vi "Magazine control.vi"(0 "Intake power":dbl, 1 "Magazine power":dbl, 2 "Magazine Recovery Power":dbl, 3 "Magazine Intake power":dbl, 4 "Flywheel power":dbl, 5 "Idle flywheel power":dbl, 7 "Intake sensor":bool, 8 "Intake":bool, 10 "Shoot":bool, 11 "Outtake sensor":bool, 12 "Emergency force state":T1(ring)=enum."Nil", 13 "Initial state":T1(ring)=enum."Idle") -> (14 "Intake":dbl, 15 "Magazine":dbl, 18 "Flywheel":dbl)   [LabVIEW 2019]
panel:
  out "State":T1(ring)=enum."I-mode tweak from intake"
  # "If both (or neither) are false, the magazine goes into the idle state."
  # "These inputs can interrupt the current state."
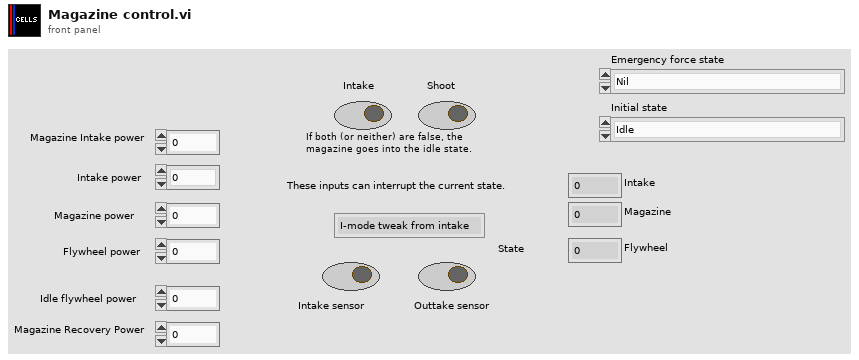
[diagram p1: front panel]
types:
  T1 = enum16{"I-mode wait for cell", "I-mode move to intake", "I-mode tweak from intake", "I-mode move cells in", "Idle", "O-mode move to outtake", "O-mode wait to shoot", "Recover from full magazine", "O-mode shoot", "Nil", "O-mode move to outtake w/o shoot"}
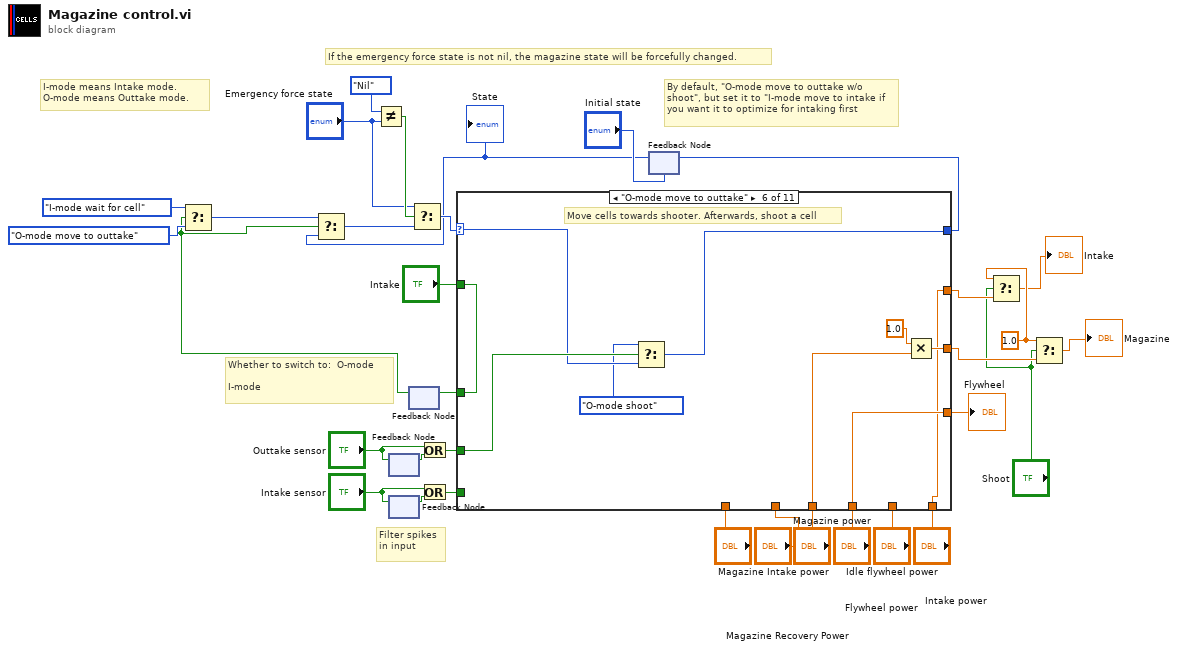
[diagram p0: block diagram]
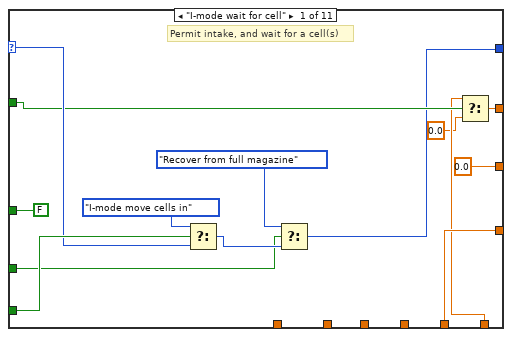
[diagram p2: hidden frame]
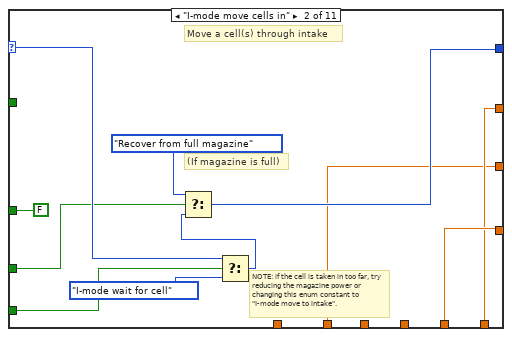
[diagram p3: hidden frame]
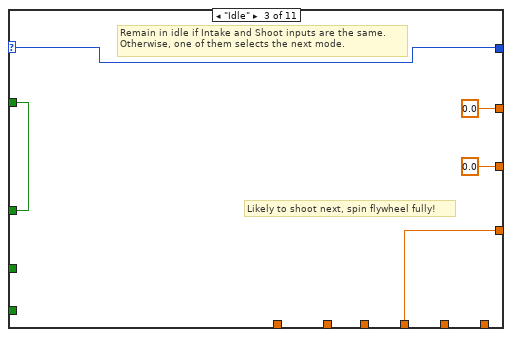
[diagram p4: hidden frame]
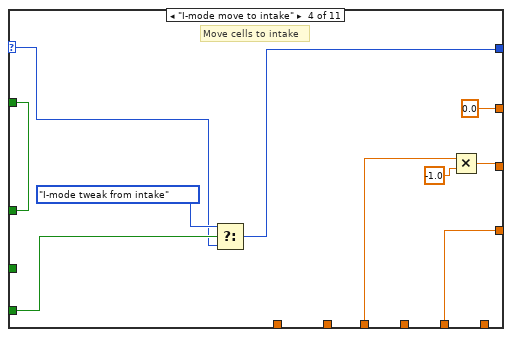
[diagram p5: hidden frame]
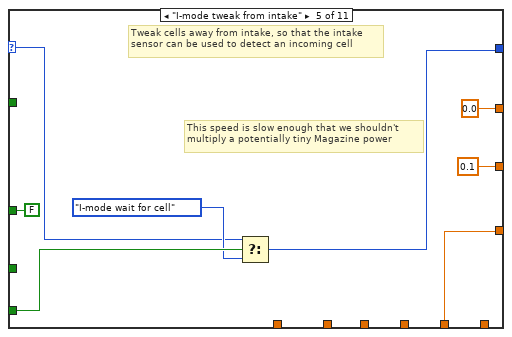
[diagram p6: hidden frame]
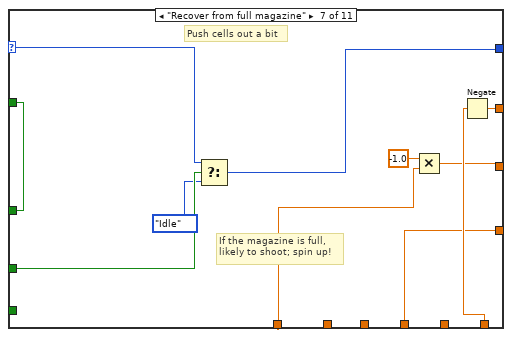
[diagram p7: hidden frame]
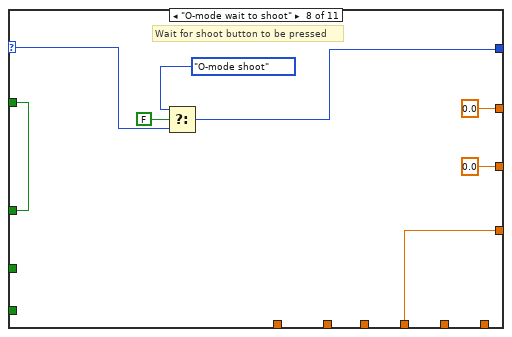
[diagram p8: hidden frame]
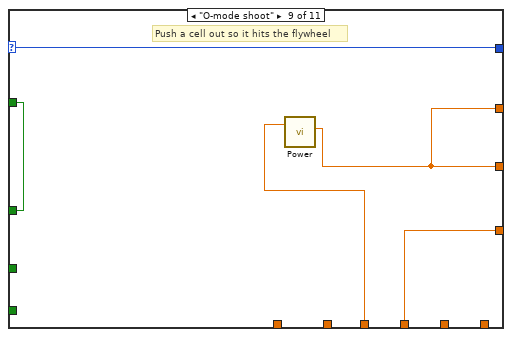
[diagram p9: hidden frame]
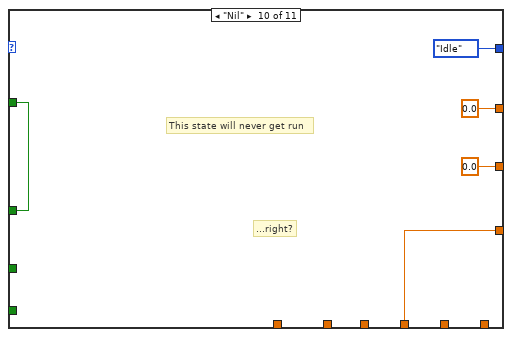
[diagram p10: hidden frame]
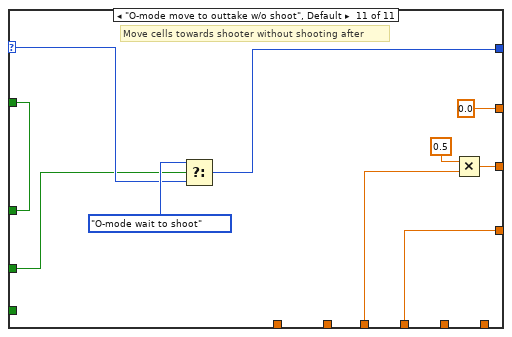
[diagram p11: hidden frame]
diagram:
  w3 = 1.0 ("t")
  # "By default, \"O-mode move to outtake w/o shoot\", but set it to \"I-mode move to intake if you want it to optimize for intaking first"
  # "Filter spikes in input"
  # "If the emergency force state is not nil, the magazine state will be forcefully changed."
  # "Whether to switch to:  O-mode\n\nI-mode"
  # "I-mode means Intake mode.\nO-mode means Outtake mode."
  n1 = Not Equal?(x=T1."Nil", y="Emergency force state") -> (x != y?=w19:bool)
  n2 = feedback #1() -> (w13:bool)  [unwired: 1 in]
  n3 = feedback-in #1("Outtake sensor") -> ()
  n4 = feedback-in #2("Intake sensor") -> ()
  n5 = feedback #2() -> (w15:bool)  [unwired: 1 in]
  n6 = feedback #3() -> (w7:bool)  [unwired: 1 in]
  n7 = Select(t=T1."I-mode wait for cell", s=w7, f=T1."O-mode move to outtake") -> (s? t:f=w25:T1)
  n8 = Or(x="Outtake sensor", y=w13) -> (x .or. y?=w12:bool)
  n9 = Or(x="Intake sensor", y=w15) -> (x .or. y?=w16:bool)
  n10 = feedback #4("Initial state") -> (w10:T1)
  "State" <- w10
  n11 = Select(t=w25, s=w7, f=w10) -> (s? t:f=w22:T1)
  n12 = Select(t="Emergency force state", s=w19, f=w22) -> (s? t:f=w21:T1)
  n13 = case shown="\"O-mode move to outtake\"" w21 {
    selector: w21 -> [w46 w57 w60 w66 w76 w85 w97 w107 w113 _ w128]
    tunnel: w16 -> [w47 w58 _ w73 w81 _ _ _ _ _ _]
    tunnel: w12 -> [w35 w50 _ _ _ w87 w98 _ _ _ w127]
    tunnel: "Magazine power" -> [_ _ _ w71 _ w89 _ _ w111 _ w125]
    tunnel: [0.0 ("Magazine") w48 0.0 ("Magazine") w69 0.1 ("Magazine") w90 w100 0.0 ("Magazine") w112 0.0 ("Magazine") w123] -> w6
    tunnel: [w42 w52 0.0 ("Intake power") 0.0 ("Intake power") 0.0 ("Intake power") w82 w102 0.0 ("Intake power") w112 0.0 ("Intake power") 0.0 ("Intake power")] -> w4
    tunnel: [w43 w53 w59 w67 w78 w91 w94 w110 w115 w116 w124] -> w33
    tunnel: "Idle flywheel power" -> [w43 w53 _ w67 w78 _ _ _ _ _ _]
    tunnel: "Intake power" -> [w40 w52 _ _ _ w82 w101 _ _ _ _]
    tunnel: "Flywheel power" -> [_ _ w59 _ _ w91 w94 w110 w115 w116 w124]
    tunnel: [w34 w51 w60 w65 w77 w86 w96 w106 w113 T1."Idle" w121] -> w28
    tunnel: "Intake" -> [w41 _ w61 w64 _ w83 w92 w104 w114 w120 w126]
    tunnel: [FALSE ("Intake") FALSE ("Intake") w61 w64 FALSE ("Intake") w83 w92 w104 w114 w120 w126] -> w26
    tunnel: "Magazine Intake power" -> [_ w48 _ _ _ _ _ _ _ _ _]
    tunnel: "Magazine Recovery Power" -> [_ _ _ _ _ _ w93 _ _ _ _]
    frame "I-mode wait for cell" {
      # "Permit intake, and wait for a cell(s)"
      n14 = Select(t=T1."I-mode move cells in", s=w47, f=w46) -> (s? t:f=w37:T1)
      n15 = Select(t=T1."Recover from full magazine", s=w35, f=w37) -> (s? t:f=w34:T1)
      n16 = Select(t=w40, s=w41, f=0.0) -> (s? t:f=w42:dbl)
    }
    frame "I-mode move cells in" {
      # "NOTE: if the cell is taken in too far, try reducing the magazine power or changing this enum constant to \"I-mode move to intake\"."
      # "(If magazine is full)"
      # "Move a cell(s) through intake"
      n17 = Select(t=w57, s=w58, f=T1."I-mode wait for cell") -> (s? t:f=w55:T1)
      n18 = Select(t=T1."Recover from full magazine", s=w50, f=w55) -> (s? t:f=w51:T1)
    }
    frame "Idle" {
      # "Likely to shoot next, spin flywheel fully!"
      # "Remain in idle if Intake and Shoot inputs are the same.\nOtherwise, one of them selects the next mode."
    }
    frame "I-mode move to intake" {
      # "Move cells to intake"
      n19 = Select(t=T1."I-mode tweak from intake", s=w73, f=w66) -> (s? t:f=w65:T1)
      n20 = Multiply(x=w71, y=-1.0) -> (x*y=w69:dbl)
    }
    frame "I-mode tweak from intake" {
      # "This speed is slow enough that we shouldn't multiply a potentially tiny Magazine power"
      # "Tweak cells away from intake, so that the intake sensor can be used to detect an incoming cell"
      n21 = Select(t=w76, s=w81, f=T1."I-mode wait for cell") -> (s? t:f=w77:T1)
    }
    frame "O-mode move to outtake" {
      # "Move cells towards shooter. Afterwards, shoot a cell"
      n22 = Select(t=T1."O-mode shoot", s=w87, f=w85) -> (s? t:f=w86:T1)
      n23 = Multiply(x=1.0, y=w89) -> (x*y=w90:dbl)
    }
    frame "Recover from full magazine" {
      # "If the magazine is full, likely to shoot; spin up!"
      # "Push cells out a bit"
      n24 = Select(t=w97, s=w98, f=T1."Idle") -> (s? t:f=w96:T1)
      n25 = Multiply(x=-1.0, y=w93) -> (x*y=w100:dbl)
      n26 = Negate(x=w101) -> (-x=w102:dbl)
    }
    frame "O-mode wait to shoot" {
      # "Wait for shoot button to be pressed"
      n27 = Select(t=T1."O-mode shoot", s=FALSE, f=w107) -> (s? t:f=w106:T1)
    }
    frame "O-mode shoot" {
      # "Push a cell out so it hits the flywheel"
      n28 = call "Power.vi"("Positive Power"=w111) -> ("Output"=w112:dbl)  [unwired: 10 in]
    }
    frame "Nil" {
      # "...right?"
      # "This state will never get run"
    }
    frame "O-mode move to outtake w/o shoot", Default {
      # "Move cells towards shooter without shooting after"
      n29 = Select(t=T1."O-mode wait to shoot", s=w127, f=w128) -> (s? t:f=w121:T1)
      n30 = Multiply(x=0.5, y=w125) -> (x*y=w123:dbl)
    }
  }
  "Flywheel" <- w33
  n31 = feedback-in #3(w26) -> ()
  n32 = feedback-in #4(w28) -> ()
  n33 = Select(t=w3, s="Shoot", f=w4) -> (s? t:f=→"Intake":dbl)
  n34 = Select(t=w3, s="Shoot", f=w6) -> (s? t:f=→"Magazine":dbl)
